vi "ConfigParseInitialConfiguration.vi"(8 "error in (no error)":errorcluster, 11 "Root Refnum in":refnum<k20>) -> (0 "error out":errorcluster, 3 "Configuration Array":string[][](array[string]))   [LabVIEW 2018]
uses:
  <vilib>/xml/NI_XML.lvlib
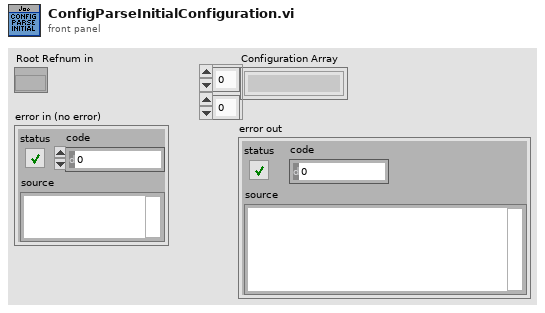
[diagram p1: front panel]
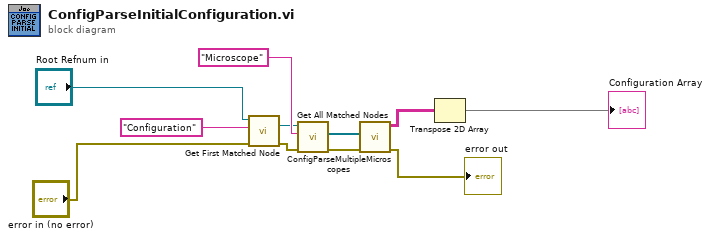
[diagram p0: block diagram]
diagram:
  n1 = call <vilib>:"Get First Matched Node.vi"("error in (no error)"="error in (no error)", "XPath expression"="Configuration" ("Get Elements By Tag Name"), "node in"="Root Refnum in") -> ("error out"=w3:errorcluster, "node result"=w4:refnum<k20>)  [unwired: 6 in, 1 out]
  n2 = call <vilib>:"Get All Matched Nodes.vi"("error in (no error)"=w3, "XPath expression"="Microscope", "node in"=w4) -> ("error out"=w5:errorcluster, "node result array"=w6:refnum<k20>[])  [unwired: 6 in, 1 out]
  n3 = call "ConfigParseMultipleMicroscopes.vi"("error in (no error)"=w5, "node result array"=w6) -> ("error out"=→"error out":errorcluster, "Array"=w9:string[][])  [unwired: 8 in]
  n4 = Transpose 2D Array(2D array=w9) -> (transposed array=→"Configuration Array":string[][])
